vi "10000개의 난수 정렬.vi"() -> ()   [LabVIEW 2019]
panel:
  out "Sum":i32
  out "Waveform Graph":i32[](graph)
  out "Numeric 6":i32
  out "Numeric 5":i32
  out "Numeric 4":i32
  out "Numeric 3":i32
  out "Numeric 2":i32
  out "Numeric":i32
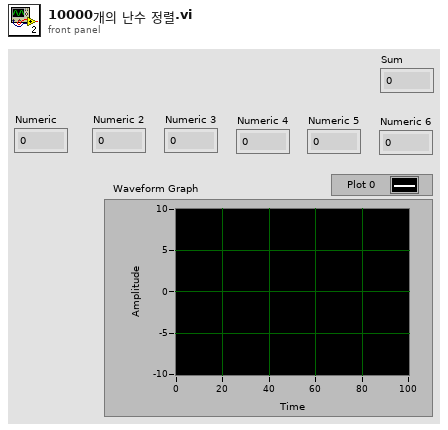
[diagram p1: front panel]
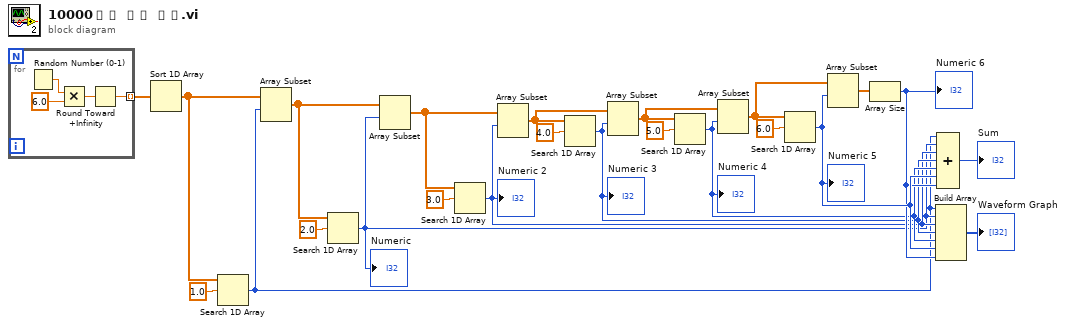
[diagram p0: block diagram]
diagram:
  n1 = for {
    tunnel: [w24] -> w23 mode=indexing
    n2 = Random Number (0-1)() -> (number: 0 to 1=w26:dbl)
    n3 = Multiply(x=w26, y=6.0) -> (x*y=w25:dbl)
    n4 = Round Toward +Infinity(x=w25) -> (ceil(x): smallest int >= x=w24:dbl)
  }
  n5 = Sort 1D Array(array=w23) -> (sorted array=w22:dbl[])
  n6 = Search 1D Array(1D array=w22, element=1.0) -> (index of element=w3:i32)  [unwired: 1 in]
  n7 = Array Subset(array=w22, index=w3) -> (w21:dbl[])  [unwired: 1 in]
  n8 = Search 1D Array(1D array=w21, element=2.0) -> (index of element=w4:i32)  [unwired: 1 in]
  "Numeric" <- w4
  n9 = Array Subset(array=w21, index=w4) -> (w20:dbl[])  [unwired: 1 in]
  n10 = Search 1D Array(1D array=w20, element=3.0) -> (index of element=w5:i32)  [unwired: 1 in]
  "Numeric 2" <- w5
  n11 = Array Subset(array=w20, index=w5) -> (w19:dbl[])  [unwired: 1 in]
  n12 = Search 1D Array(1D array=w19, element=4.0) -> (index of element=w6:i32)  [unwired: 1 in]
  "Numeric 3" <- w6
  n13 = Array Subset(array=w19, index=w6) -> (w18:dbl[])  [unwired: 1 in]
  n14 = Search 1D Array(1D array=w18, element=5.0) -> (index of element=w7:i32)  [unwired: 1 in]
  "Numeric 4" <- w7
  n15 = Array Subset(array=w18, index=w7) -> (w17:dbl[])  [unwired: 1 in]
  n16 = Search 1D Array(1D array=w17, element=6.0) -> (index of element=w10:i32)  [unwired: 1 in]
  "Numeric 5" <- w10
  n17 = Array Subset(array=w17, index=w10) -> (w9:dbl[])  [unwired: 1 in]
  n18 = Array Size(array=w9) -> (size(s)=w8:i32)
  "Numeric 6" <- w8
  n19 = Build Array(w3, w4, w5, w6, w7, w10, w8) -> (→"Waveform Graph":i32[])
  n20 = Compound Arithmetic op=ADD(w3, w4, w5, w6, w7, w10, w8) -> (→"Sum":i32)
